vi "Shutdown.vi"(8 "Error In":errorcluster) -> (0 "Error Out":errorcluster)   [LabVIEW 2014, in "Logger.lvlib"]
uses:
  Logger.lvlib
  Private/_Logger Action.ctl
  Private/File/_Action.ctl
  Private/Error/_Action.ctl
  Private/File/File.lvlib
  Private/Error/Error.lvlib
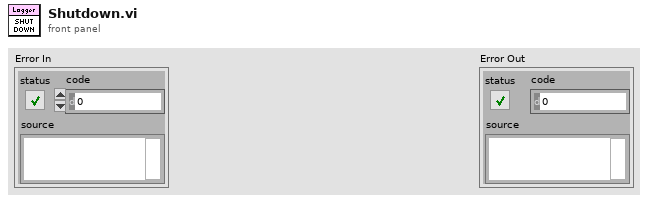
[diagram p1: front panel]
types:
  T1 = typedef "Logger.lvlib/File.lvlib/_Action.ctl" = enum16{"Initialize", "Set File Size Limit", "Set Root Folder", "Set Application Name", "Start", "Write", "Stop", "Shutdown"}
  T2 = typedef "Logger.lvlib/Error.lvlib/_Action.ctl" = enum16{"Initialize", "Get", "Set Verbosity", "Set User-Defined Codes", "Set User-Defined Descriptions", "Shutdown"}
  T3 = typedef "Logger.lvlib/_Logger Action.ctl" = enum16{"Initialize", "Register", "Log", "Unregister", "Set Level", "Shutdown"}
  T4 = typedef "LV-Logger.lvlib/Message.ctl" = cluster{"Time Stamp":timestamp, "Tag":T5, "Source":string, "Text":string}
  T5 = typedef "LV-Logger.lvlib/Tag.ctl" = enum16{"Fatal", "Error", "Warn", "Info", "Debug", "Trace"}
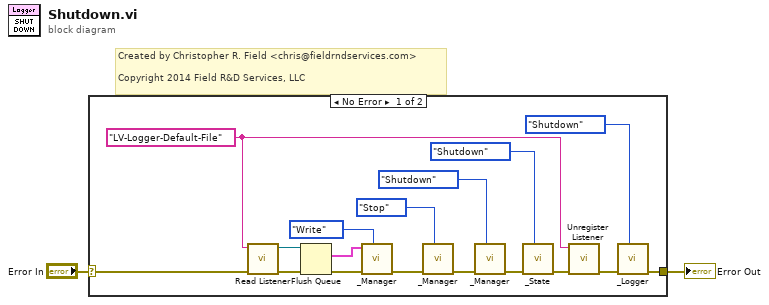
[diagram p0: block diagram]
diagram:
  # "Created by Christopher R. Field <chris@fieldrndservices.com>\n\nCopyright 2014 Field R&D Services, LLC"
  n1 = case shown="No Error" "Error In" {
    selector: "Error In" -> [w14 w20]
    tunnel: [w18 w20] -> w1
    frame No Error {
      w8 = "LV-Logger-Default-File" ("Listener ID")
      n2 = call "Read Listener.vi"("Error In"=w14, "Listener ID"=w8) -> ("Error Out"=w12:errorcluster, "Listener"=w13:refnum<queue>)  [unwired: 8 in]
      n3 = Flush Queue(queue=w13, error in (no error)=w12) -> (remaining elements=w10:T4[], error out=w9:errorcluster)  [unwired: 1 out]
      n4 = call "_Manager.vi"("Action"=_Action."Write", "Error In"=w9, "Set Value"=w10) -> ("Error Out"=w7:errorcluster)  [unwired: 8 in]
      n5 = call "_Manager.vi"("Action"=_Action."Stop", "Error In"=w7) -> ("Error Out"=w5:errorcluster)  [unwired: 9 in]
      n6 = call "_Manager.vi"("Action"=_Action."Shutdown", "Error In"=w5) -> ("Error Out"=w4:errorcluster)  [unwired: 9 in]
      n7 = call "_State.vi"("Action"=_Action."Shutdown", "Error In"=w4) -> ("Error Out"=w3:errorcluster)  [unwired: 8 in, 1 out]
      n8 = call "Unregister Listener.vi"("Error In"=w3, "Listener ID"=w8) -> ("Error Out"=w17:errorcluster)  [unwired: 9 in]
      n9 = call "_Logger.vi"("Action"=_Logger_Action."Shutdown", "Error In"=w17) -> ("Error Out"=w18:errorcluster)  [unwired: 9 in]
    }
    frame Error {
    }
  }
  "Error Out" <- w1
